vi "Fire Data Changed.vi"(8 "error in (no error)":errorcluster, 11 "Data in":refnum<class "Data.lvclass">) -> (0 "error out":errorcluster, 3 "Data out":refnum<class "Data.lvclass">)   [LabVIEW 2017, in "Filled Text Fields Actor.lvlib" / "Data.lvclass"]
uses:
  Data.lvclass
  Data.PrivateData.ctl
  Data.lvclass/Data.ctl
  getData.vi
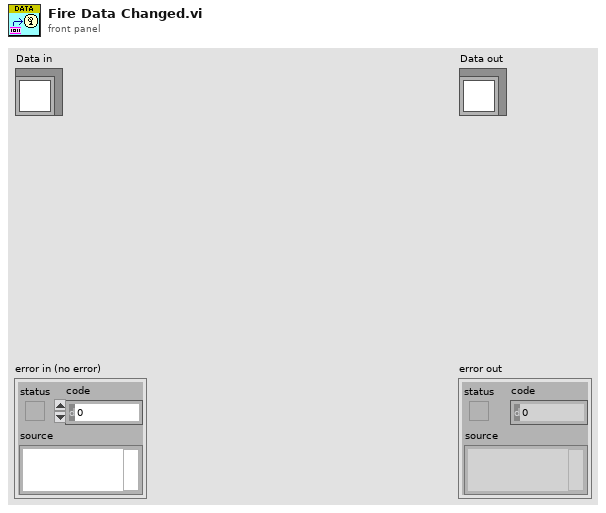
[diagram p1: front panel]
types:
  T1 = typedef "Filled Text Fields Actor.lvlib/Data.lvclass/Data.PrivateData.ctl" = cluster{"Data":string}
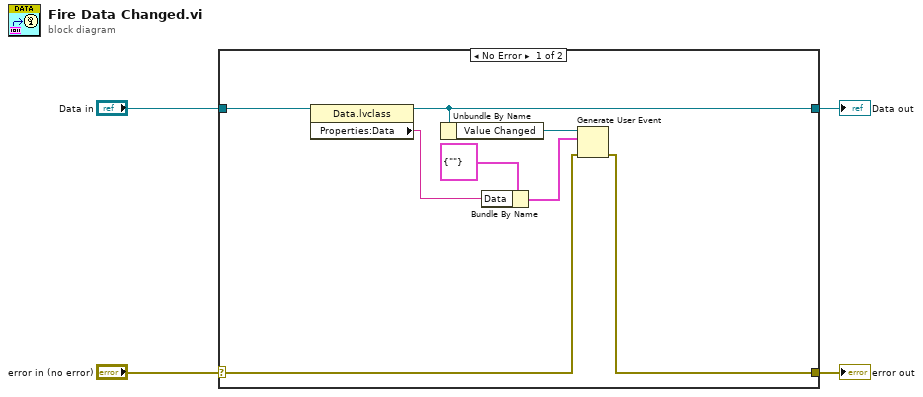
[diagram p0: block diagram]
diagram:
  n1 = case shown="No Error" "error in (no error)" {
    selector: "error in (no error)" -> [w6 w14]
    tunnel: [w5 w14] -> w3
    tunnel: [w11 w13] -> w1
    tunnel: "Data in" -> [w12 w13]
    frame No Error {
      n2 = property class="Data.lvclass"(reference=w12) -> (reference out=w11:refnum<class "Data.lvclass">, "Properties:Data"=w8:string)  [unwired: 1 in, 1 out]
      n3 = Unbundle By Name(w11) -> ("Value Changed"=w10:refnum<user-event>)
      n4 = Bundle By Name(cluster=T1 {"Data"=""} ("Private Data"), "Data"=w8) -> (w7:T1)
      n5 = Generate User Event(user event=w10, event data cluster=w7, error in=w6) -> (error out=w5:errorcluster)  [unwired: 1 in, 1 out]
    }
    frame Error {
    }
  }
  "error out" <- w3
  "Data out" <- w1
